vi "Unit Test.vi"() -> ()   [LabVIEW 2016, in "Instrument.OxfordVRM.lvclass"]
uses:
  Instrument.OxfordVRM.lvclass
  <vilib>/addons/_JKI Toolkits/Caraya/classes/Test/Test.lvclass
panel:
  out "Status 3":string
  out "Status 2":string
  out "Status":string
  out "error out":errorcluster
  out "Instrument.OxfordVRM out":refnum<class "Instrument.OxfordVRM.lvclass">
  in  "Instrument.OxfordVRM in":refnum<class "Instrument.OxfordVRM.lvclass">
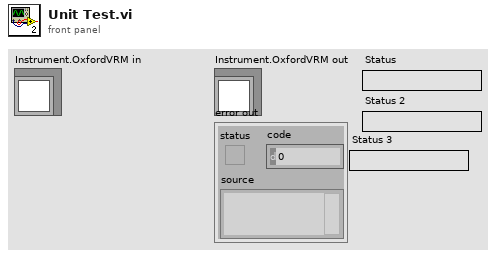
[diagram p1: front panel]
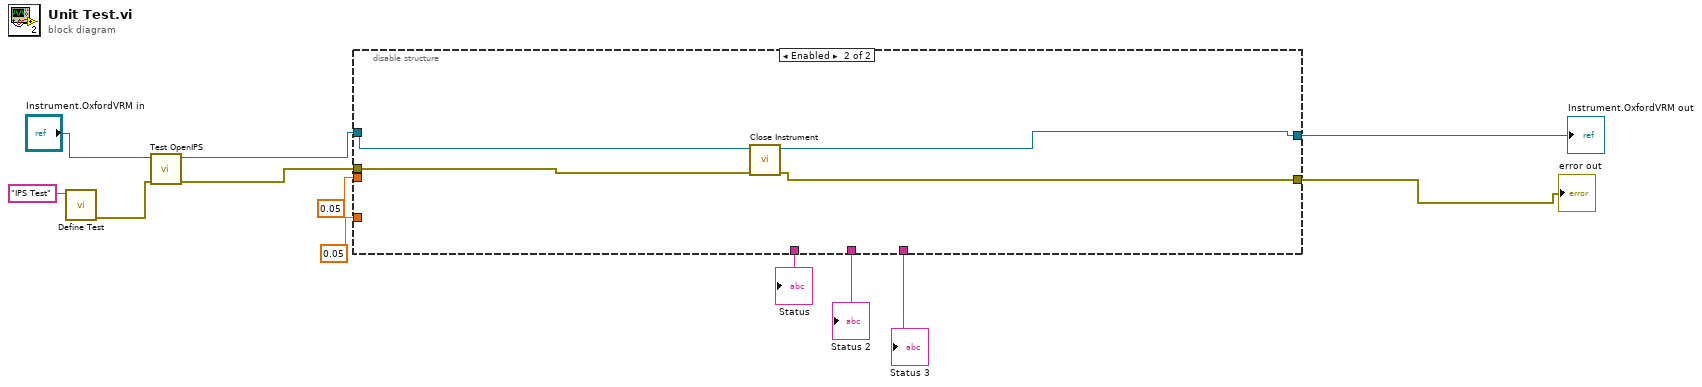
[diagram p0: block diagram]
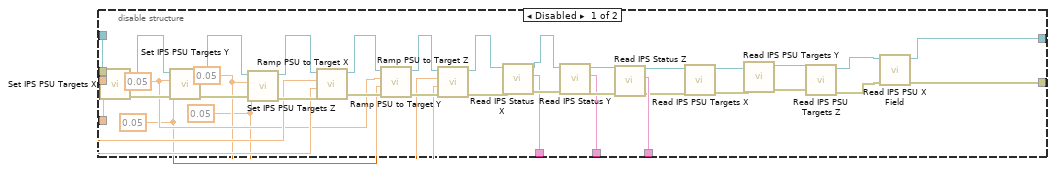
[diagram p2: hidden frame]
diagram:
  n1 = call <vilib>:"Define Test.vi"("Label (VI Title)"="IPS Test") -> ("error out"=w2:errorcluster)  [unwired: 10 in]
  n2 = call "Test OpenIPS.vi"("error in (no error)"=w2, "Instrument.OxfordVRM in"="Instrument.OxfordVRM in") -> ("error out"=w3:errorcluster, "Instrument.OxfordVRM out"=w11:refnum<class "Instrument.OxfordVRM.lvclass">)  [unwired: 8 in]
  n3 = disable-structure "Diagram Disable Structure" shown="Enabled" {
    disable-tunnel: w11 -> [w49 w53]
    disable-tunnel: 0.05 ("Target Field (T)") -> [w32 _]
    disable-tunnel: 0.05 ("Target Field Rate (T/min)") -> [w31 _]
    disable-tunnel: [w26 _] -> w8
    disable-tunnel: [w25 _] -> w7
    disable-tunnel: [w24 _] -> w6
    disable-tunnel: [w15 w51] -> w5
    disable-tunnel: [w13 w52] -> w4
    disable-tunnel: w3 -> [_ w50]
    frame Disabled {
      w27 = 0.05 ("Target Field Rate (T/min)")
      w28 = 0.05 ("Target Field (T)")
      w29 = 0.05 ("Target Field Rate (T/min)")
      w30 = 0.05 ("Target Field (T)")
      n4 = call "Set IPS PSU Targets X.vi"("Target Field Rate (T/min)"=w31, "Target Field (T)"=w32, "Instrument.OxfordVRM in"=w49) -> ("error out"=w41:errorcluster, "Instrument.OxfordVRM out"=w42:refnum<class "Instrument.OxfordVRM.lvclass">, "error in (no error)"=w14:errorcluster)  [unwired: 5 in, 1 out]
      n5 = call "Set IPS PSU Targets Y.vi"("error in (no error)"=w41, "Target Field Rate (T/min)"=w29, "Target Field (T)"=w30, "Instrument.OxfordVRM in"=w42) -> ("error out"=w40:errorcluster, "Instrument.OxfordVRM out"=w43:refnum<class "Instrument.OxfordVRM.lvclass">)  [unwired: 5 in, 1 out]
      n6 = call "Set IPS PSU Targets Z.vi"("error in (no error)"=w40, "Target Field Rate (T/min)"=w27, "Target Field (T)"=w28, "Instrument.OxfordVRM in"=w43) -> ("error out"=w39:errorcluster, "Instrument.OxfordVRM out"=w44:refnum<class "Instrument.OxfordVRM.lvclass">)  [unwired: 5 in, 1 out]
      n7 = call "Ramp PSU to Target X.vi"("error in (no error)"=w39, "Target Rate (T/min)"=w31, "Target Field (T)"=w32, "Instrument.OxfordVRM in"=w44) -> ("error out"=w38:errorcluster, "Instrument.OxfordVRM out"=w45:refnum<class "Instrument.OxfordVRM.lvclass">)  [unwired: 6 in]
      n8 = call "Ramp PSU to Target Y.vi"("error in (no error)"=w38, "Target Rate (T/min)"=w29, "Target Field (T)"=w30, "Instrument.OxfordVRM in"=w45) -> ("error out"=w37:errorcluster, "Instrument.OxfordVRM out"=w46:refnum<class "Instrument.OxfordVRM.lvclass">)  [unwired: 6 in]
      n9 = call "Ramp PSU to Target Z.vi"("error in (no error)"=w37, "Target Rate (T/min)"=w27, "Target Field (T)"=w28, "Instrument.OxfordVRM in"=w46) -> ("error out"=w36:errorcluster, "Instrument.OxfordVRM out"=w47:refnum<class "Instrument.OxfordVRM.lvclass">)  [unwired: 6 in]
      n10 = call "Read IPS Status X.vi"("error in (no error)"=w36, "Instrument.OxfordVRM in"=w47) -> ("error out"=w35:errorcluster, "Status"=w26:string, "Instrument.OxfordVRM out"=w48:refnum<class "Instrument.OxfordVRM.lvclass">)  [unwired: 7 in]
      n11 = call "Read IPS Status Y.vi"("error in (no error)"=w35, "Instrument.OxfordVRM in"=w48) -> ("error out"=w33:errorcluster, "Status"=w25:string, "Instrument.OxfordVRM out"=w34:refnum<class "Instrument.OxfordVRM.lvclass">)  [unwired: 7 in]
      n12 = call "Read IPS Status Z.vi"("error in (no error)"=w33, "Instrument.OxfordVRM in"=w34) -> ("error out"=w20:errorcluster, "Status"=w24:string, "Instrument.OxfordVRM out"=w23:refnum<class "Instrument.OxfordVRM.lvclass">)  [unwired: 7 in]
      n13 = call "Read IPS PSU Targets X.vi"("error in (no error)"=w20, "Instrument.OxfordVRM in"=w23) -> ("error out"=w19:errorcluster, "Instrument.OxfordVRM out"=w22:refnum<class "Instrument.OxfordVRM.lvclass">)  [unwired: 6 in, 2 out]
      n14 = call "Read IPS PSU Targets Y.vi"("error in (no error)"=w19, "Instrument.OxfordVRM in"=w22) -> ("error out"=w18:errorcluster, "Instrument.OxfordVRM out"=w21:refnum<class "Instrument.OxfordVRM.lvclass">)  [unwired: 6 in, 2 out]
      n15 = call "Read IPS PSU Targets Z.vi"("error in (no error)"=w18, "Instrument.OxfordVRM in"=w21) -> ("error out"=w16:errorcluster, "Instrument.OxfordVRM out"=w17:refnum<class "Instrument.OxfordVRM.lvclass">)  [unwired: 6 in, 2 out]
      n16 = call "Read IPS PSU X Field.vi"("error in (no error)"=w16, "Instrument.OxfordVRM in"=w17) -> ("error out"=w15:errorcluster, "Instrument.OxfordVRM out"=w13:refnum<class "Instrument.OxfordVRM.lvclass">)  [unwired: 7 in, 1 out]
    }
    frame Enabled {
      n17 = call-dynamic "Close Instrument.vi"("error in (no error)"=w50, "Instrument.OxfordVRM in"=w53) -> ("error out"=w51:errorcluster, "Instrument.OxfordVRM out"=w52:refnum<class "Instrument.OxfordVRM.lvclass">)  [unwired: 8 in]
    }
  }
  "Instrument.OxfordVRM out" <- w4
  "error out" <- w5
  "Status" <- w8
  "Status 2" <- w7
  "Status 3" <- w6
